vi "ble_discover_handle_table.vi"(6 "Connection Status":T1={"MAC Address"="", "cnx handle"=0, "cnx flags"=0, "Address Type"=125, "Connection Interval (ms)"=125, "Timeout(ms)"=125, "Latency"=0, "bonding handle"=0} {"Address Type" items=["Public", "Random"]}, 8 "error in (no error)":errorcluster, 11 "COM Bluegiga in":refnum<visa-resource-name>) -> (0 "error out":errorcluster, 2 "Handle table":string[][](array[string]), 3 "COM Bluegiga out":refnum<visa-resource-name>)   [LabVIEW 2013]
uses:
  type_def/connection_status_bundle.ctl
  type_def/address_type.ctl
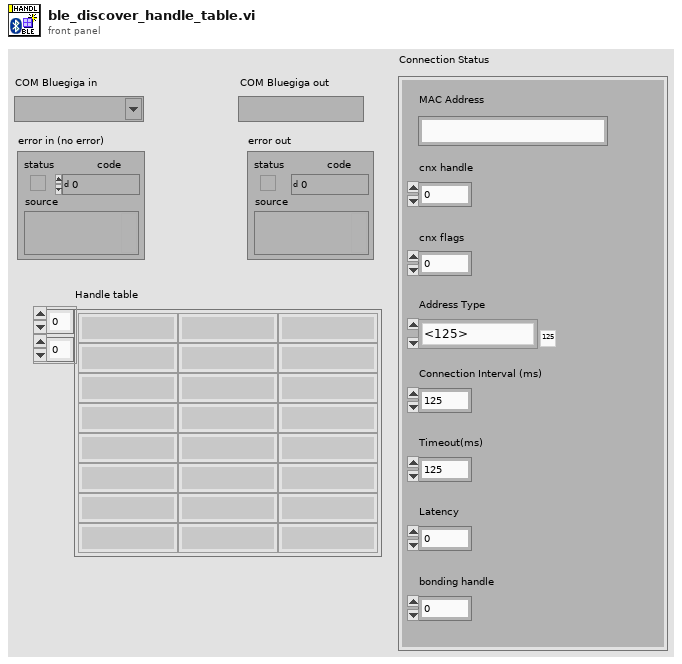
[diagram p1: front panel]
types:
  T1 = typedef "connection_status_bundle.ctl" = cluster{"MAC Address":string, "cnx handle":u8, "cnx flags":u8, "Address Type":T2, "Connection Interval (ms)":u16, "Timeout(ms)":u16, "Latency":u16, "bonding handle":u8}
  T2 = typedef "address_type.ctl" = u8
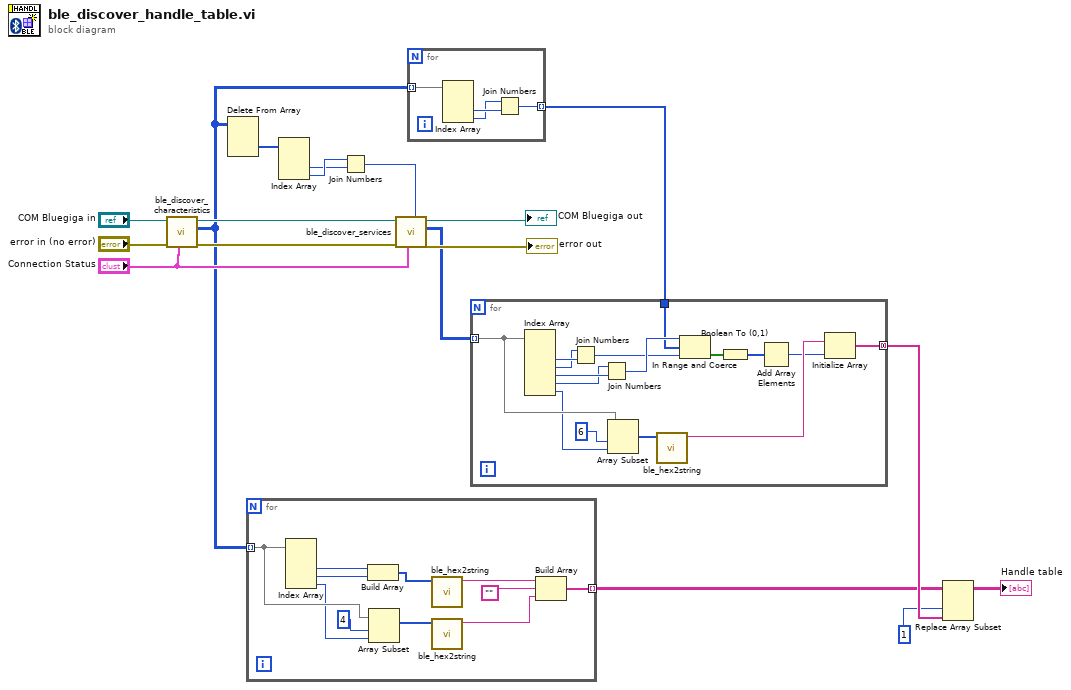
[diagram p0: block diagram]
diagram:
  n1 = call "ble_discover_characteristics.vi"("Connection Status"="Connection Status", "error in (no error)"="error in (no error)", "COM Bluegiga in"="COM Bluegiga in") -> ("error out"=w15:errorcluster, "characteristics_info"=w4:u8[][], "COM Bluegiga out"=w16:refnum<visa-resource-name>)  [unwired: 6 in]
  n2 = Delete From Array(array=w4) -> (deleted portion=w12:u8[])  [unwired: 3 in, 1 out]
  n3 = for {
    tunnel: w4 -> [w29] mode=indexing
    tunnel: [w27] -> w9 mode=indexing
    n4 = Index Array(array=w29) -> (element #2=w24:u8, element #3=w25:u8, element #4=w26:u8)  [unwired: 4 in, 1 out]
    n5 = Build Array(w24, w25) -> (w20:u8[])
    n6 = Array Subset(array=w29, index=4, length=w26) -> (w21:u8[])
    n7 = call "ble_hex2string.vi"("Byte Array IN (index0 LS byte)"=w20) -> ("HEX string OUT"=w19:string)  [unwired: 10 in]
    n8 = call "ble_hex2string.vi"("Byte Array IN (index0 LS byte)"=w21) -> ("HEX string OUT"=w22:string)  [unwired: 10 in]
    n9 = Build Array(w19, "", w22) -> (w27:string[])
  }
  n10 = Index Array(array=w12) -> (element #2=w1:u8, element #3=w2:u8)  [unwired: 3 in, 1 out]
  n11 = Join Numbers(hi=w2, lo=w1) -> ((hi.lo)=w11:u16)
  n12 = call "ble_discover_services.vi"("Last Handle Number (0xFFFF)"=w11, "Connection Status"="Connection Status", "error in (no error)"=w15, "COM Bluegiga in"=w16) -> ("error out"=→"error out":errorcluster, "service_info"=w6:u8[][], "COM Bluegiga out"=→"COM Bluegiga out":refnum<visa-resource-name>)  [unwired: 5 in]
  n13 = for {
    tunnel: w4 -> [w33] mode=indexing
    tunnel: [w32] -> w3 mode=indexing
    n14 = Index Array(array=w33) -> (element #2=w31:u8, element #3=w30:u8)  [unwired: 3 in, 1 out]
    n15 = Join Numbers(hi=w30, lo=w31) -> ((hi.lo)=w32:u16)
  }
  n16 = for {
    tunnel: w6 -> [w49] mode=indexing
    tunnel: [w46] -> w10 mode=concatenating
    tunnel: w3 -> [w39]
    n17 = Index Array(array=w49) -> (element #2=w35:u8, element #3=w34:u8, element #4=w43:u8, element #5=w42:u8, element #6=w48:u8)  [unwired: 6 in, 1 out]
    n18 = Join Numbers(hi=w34, lo=w35) -> ((hi.lo)=w40:u16)
    n19 = Join Numbers(hi=w42, lo=w43) -> ((hi.lo)=w41:u16)
    n20 = Array Subset(array=w49, index=6, length=w48) -> (w45:u8[])
    n21 = call "ble_hex2string.vi"("Byte Array IN (index0 LS byte)"=w45) -> ("HEX string OUT"=w44:string)  [unwired: 10 in]
    n22 = In Range and Coerce(upper limit=w41, x=w39, lower limit=w40) -> (In Range?=w38:bool[])  [unwired: 1 out]
    n23 = Boolean To (0,1)(Boolean=w38) -> (0, 1=w37:i16[])
    n24 = Add Array Elements(numeric array=w37) -> (sum=w36:i16)
    n25 = Initialize Array(w44, w36) -> (w46:string[])
  }
  n26 = Replace Array Subset(array=w9, new element=w10, index (col)=1 ("disabled index (col)")) -> (→"Handle table":string[][])  [unwired: 1 in]
